vi "Untitled 4.vi"   [LabVIEW 2019]
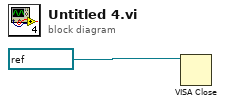
[diagram p0: block diagram]
diagram:
  n1 = VISA Close(VISA resource name=refnum<visa-resource-name> "COM4") -> ()  [unwired: 1 in, 1 out]
